vi "ReadBankChannelsNode.vi"(8 "Error In":errorcluster, 11 "Channels Node In":refnum<k20>) -> (0 "Error Out":errorcluster, 2 "Channel Names":string[](array[string]), 3 "Channels Node Out":refnum<k20>)   [LabVIEW 2012]
uses:
  <vilib>/xml/NI_XML.lvlib
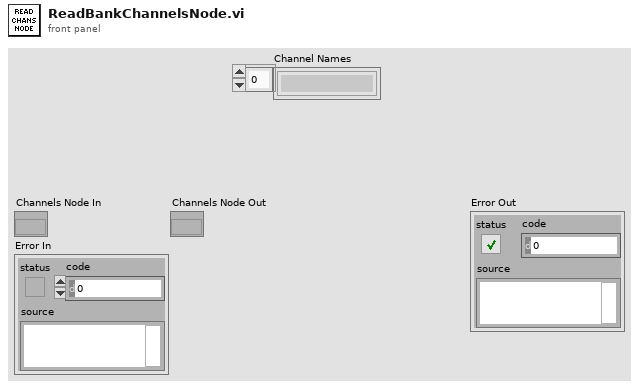
[diagram p1: front panel]
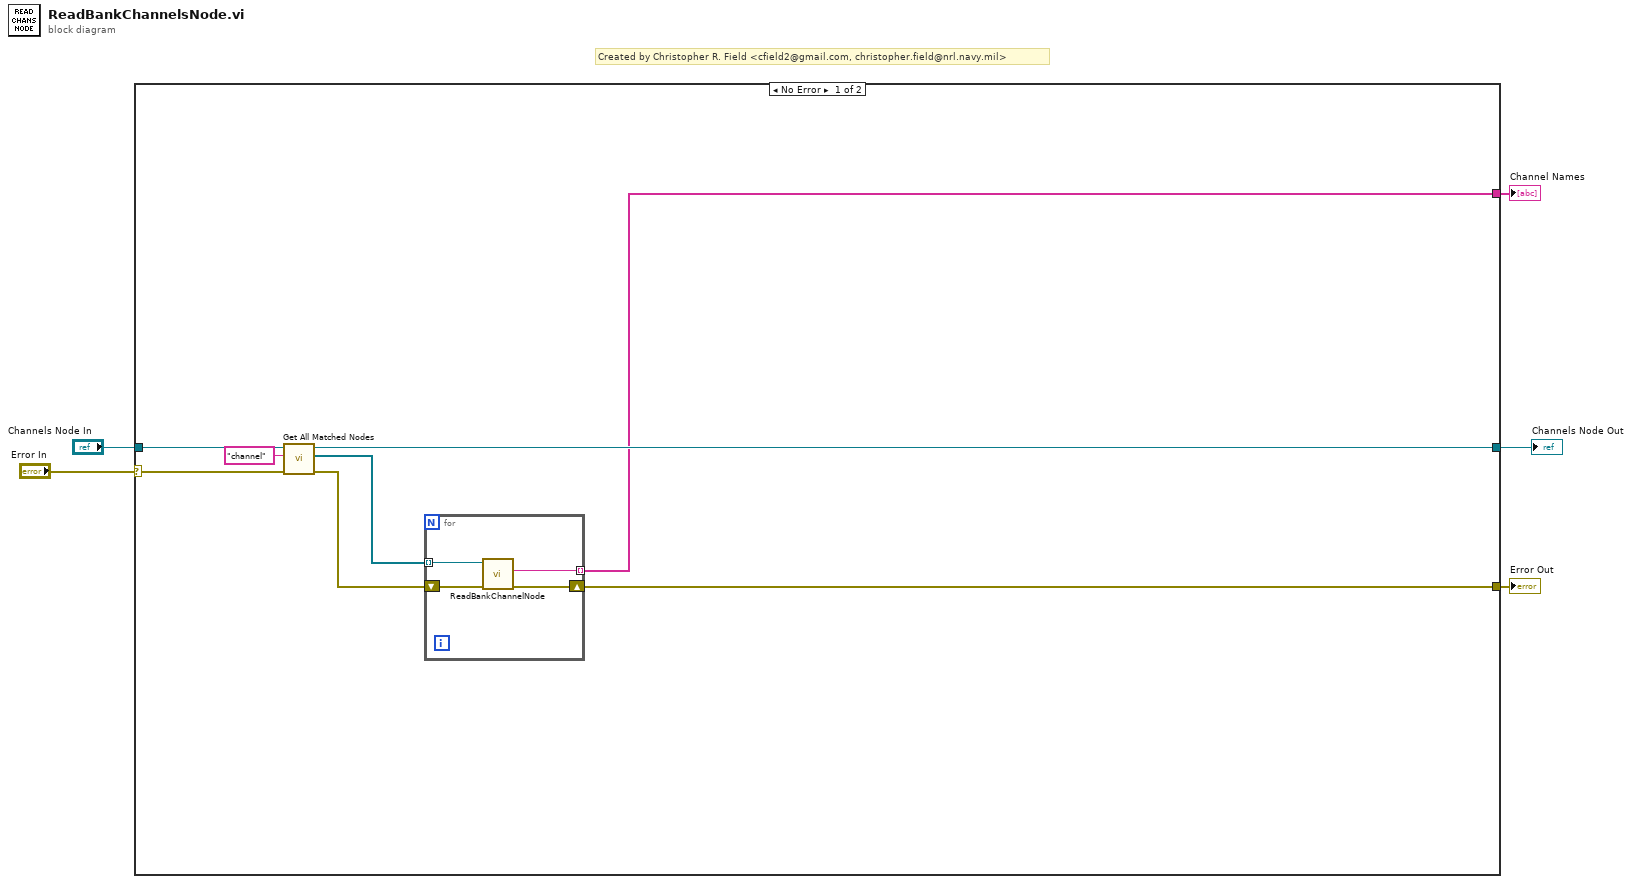
[diagram p0: block diagram]
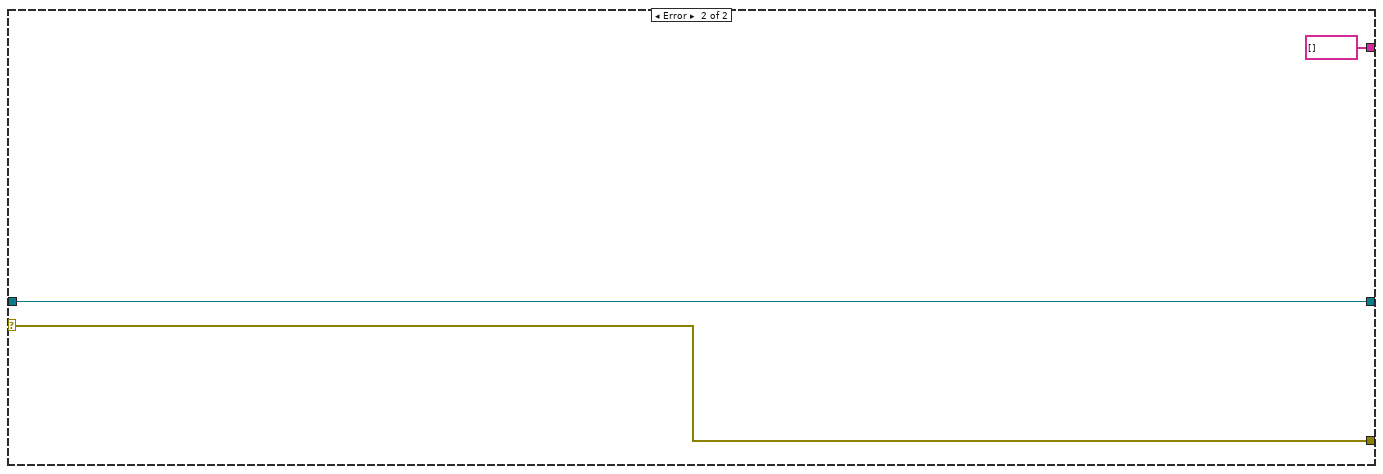
[diagram p2: hidden frame]
diagram:
  # "Created by Christopher R. Field <cfield2@gmail.com, christopher.field@nrl.navy.mil>"
  n1 = case shown="No Error" "Error In" {
    selector: "Error In" -> [w12 w19]
    tunnel: "Channels Node In" -> [w13 w20]
    tunnel: [w8 w19] -> w3
    tunnel: [w7 w20] -> w2
    tunnel: [w6 string[] []] -> w1
    frame No Error {
      n2 = call <vilib>:"Get All Matched Nodes.vi"("error in (no error)"=w12, "XPath expression"="channel", "node in"=w13) -> ("error out"=w9:errorcluster, "node result array"=w10:refnum<k20>[], "node out"=w7:refnum<k20>)  [unwired: 6 in]
      n3 = for {
        tunnel: w10 -> [w17] mode=indexing
        shift-right: [w15] -> w8
        shift-left: w9 -> [w16]
        tunnel: [w14] -> w6 mode=indexing
        n4 = call "ReadBankChannelNode.vi"("Error In"=w16, "Bank Channel Node In"=w17) -> ("Error Out"=w15:errorcluster, "Name"=w14:string)  [unwired: 7 in, 1 out]
      }
    }
    frame Error {
    }
  }
  "Error Out" <- w3
  "Channels Node Out" <- w2
  "Channel Names" <- w1
